vi "Write rotAngle.vi"(8 "error in (no error)":errorcluster, 10 "rotAngle":dbl[unit] min=0.0 max=6.283185307179586, 11 "MccRotMove in":refnum<class "MccRotMove.lvclass">) -> (0 "error out":errorcluster, 3 "MccRotMove out":refnum<class "MccRotMove.lvclass">)   [LabVIEW 2014, in "TCSDataDefinitions.lvlib" / "TCSMountControlCommand.lvlib" / "CommandsForRotatorAxis.lvlib" / "MccRotMove.lvclass"]
uses:
  MccRotMove.lvclass
  MccRotMove.lvclass/MccRotMove.ctl
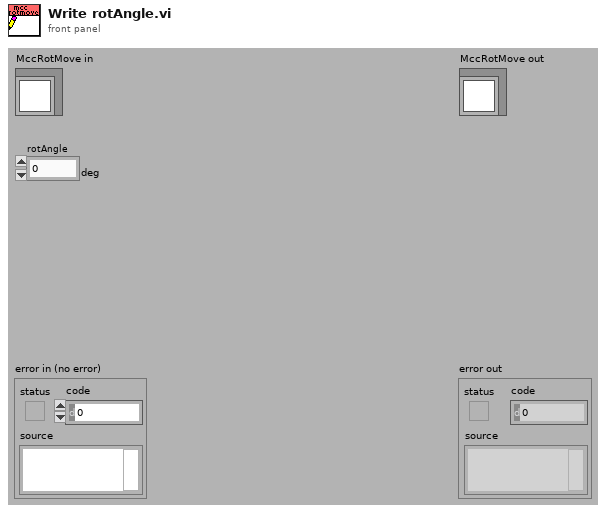
[diagram p1: front panel]
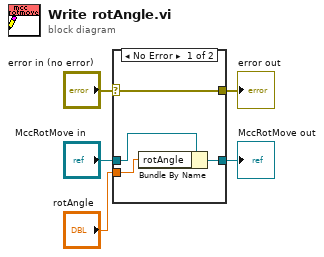
[diagram p0: block diagram]
diagram:
  n1 = case shown="No Error" "error in (no error)" {
    selector: "error in (no error)" -> [w9 w10]
    tunnel: [w9 w10] -> w4
    tunnel: [w7 w11] -> w2
    tunnel: "MccRotMove in" -> [w8 w11]
    tunnel: "rotAngle" -> [w6 _]
    frame No Error {
      n2 = Bundle By Name(cluster=w8, "rotAngle"=w6) -> (w7:refnum<class "MccRotMove.lvclass">)
    }
    frame Error {
    }
  }
  "error out" <- w4
  "MccRotMove out" <- w2
